vi "Get JSON Data.vi"(8 "error in (no error)":errorcluster, 11 "LVUnit Test Case in":refnum<class "LVUnit Test Case.lvclass">) -> (0 "error out":errorcluster, 2 "JSON Data":string, 3 "LVUnit Test Case out":refnum<class "LVUnit Test Case.lvclass">)   [LabVIEW 2017, in "LVUnit Test Case.lvclass"]
uses:
  LVUnit Test Case.lvclass
  LVUnit Test Case.lvclass/LVUnit Test Case.ctl
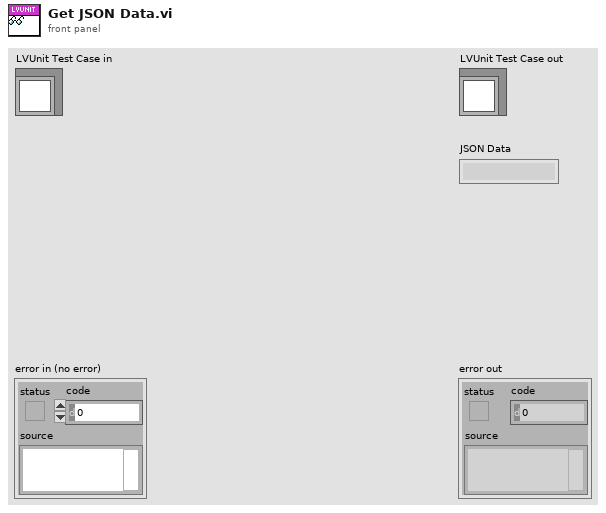
[diagram p1: front panel]
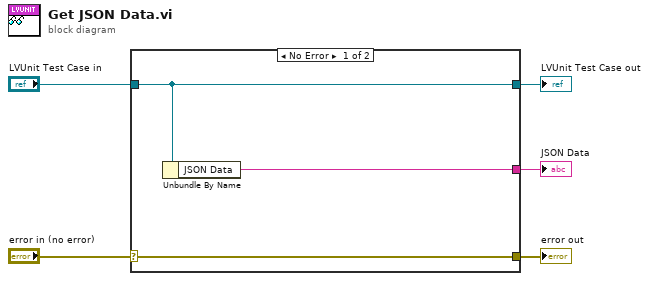
[diagram p0: block diagram]
diagram:
  n1 = case shown="No Error" "error in (no error)" {
    selector: "error in (no error)" -> [w8 w9]
    tunnel: [w8 w9] -> w4
    tunnel: [w7 w10] -> w2
    tunnel: "LVUnit Test Case in" -> [w7 w10]
    tunnel: [w6 _] -> w1
    frame No Error {
      n2 = Unbundle By Name(w7) -> ("JSON Data"=w6:string)
    }
    frame Error {
    }
  }
  "error out" <- w4
  "LVUnit Test Case out" <- w2
  "JSON Data" <- w1
